vi "DC_CNTRL_select_potential.vi"(0 "Handle":u64, 1 "Ignore NACK":bool, 2 "Read Answer?":bool, 3 "Clear  RxTx Buffer?":bool, 5 "Box Number":u16(ring), 7 "Target Potential (V)":dbl, 9 "Current Potential (V)":dbl, 11 "error in (no error)":errorcluster, 12 "Max Potential (V)":dbl) -> (4 "Handle out":u64, 15 "error out":errorcluster)   [LabVIEW 2019]
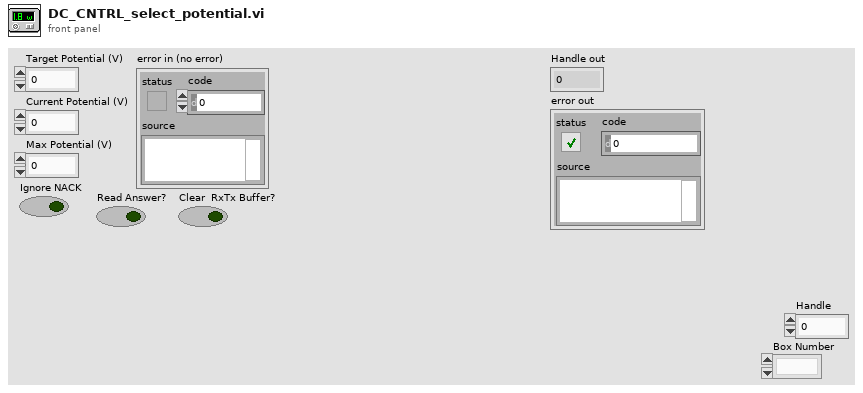
[diagram p1: front panel]
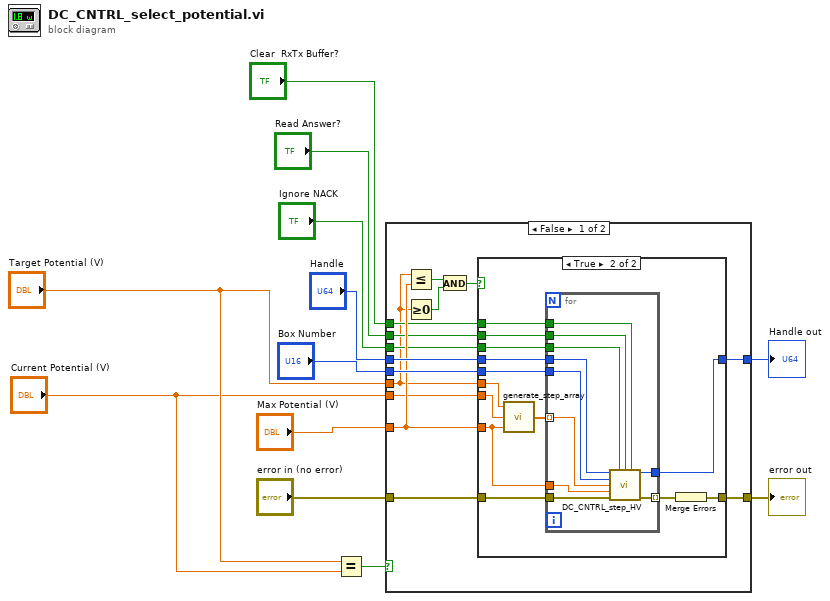
[diagram p0: block diagram]
diagram:
  n1 = Equal?(x="Target Potential (V)", y="Current Potential (V)") -> (x = y?=w12:bool)
  n2 = case shown="False" w12 {
    tunnel: "Target Potential (V)" -> [w14 _]
    tunnel: "Max Potential (V)" -> [w20 _]
    tunnel: "Handle" -> [w23 w53]
    tunnel: "Box Number" -> [w22 _]
    tunnel: "error in (no error)" -> [w21 w52]
    tunnel: "Ignore NACK" -> [w19 _]
    tunnel: "Read Answer?" -> [w18 _]
    tunnel: "Clear  RxTx Buffer?" -> [w17 _]
    tunnel: [w16 w53] -> w3
    tunnel: [w15 w52] -> w2
    tunnel: "Current Potential (V)" -> [w13 _]
    frame False {
      n3 = Less Or Equal?(x=w14, y=w20) -> (x <= y?=w25:bool)
      n4 = Greater Or Equal To 0?(x=w14) -> (x >= 0?=w24:bool)
      n5 = And(x=w25, y=w24) -> (x .and. y?=w26:bool)
      n6 = case shown="True" w26 {
        tunnel: w23 -> [w28 w41]
        tunnel: w22 -> [_ w40]
        tunnel: w21 -> [w27 w39]
        tunnel: w20 -> [_ w32]
        tunnel: w19 -> [_ w38]
        tunnel: w18 -> [_ w37]
        tunnel: w17 -> [_ w36]
        tunnel: [w28 w35] -> w16
        tunnel: [w27 w33] -> w15
        tunnel: w14 -> [_ w31]
        tunnel: w13 -> [_ w30]
        frame False {
        }
        frame True {
          n7 = call "generate_step_array.vi"("Max Potential (V)"=w32, "Current Potential (V)"=w30, "Target Potential (V)"=w31) -> ("Step Array"=w29:dbl[])
          n8 = for {
            tunnel: w41 -> [w51]
            tunnel: w40 -> [w50]
            tunnel: w39 -> [w49]
            tunnel: w32 -> [w48]
            tunnel: w38 -> [w47]
            tunnel: w37 -> [w46]
            tunnel: w36 -> [w45]
            tunnel: [w44] -> w35
            tunnel: [w43] -> w34 mode=indexing
            tunnel: w29 -> [w42] mode=indexing
            n9 = call "DC_CNTRL_step_HV.vi"("Handle"=w51, "Ignore NACK"=w47, "Read Answer?"=w46, "Clear  RxTx Buffer?"=w45, "Box Number"=w50, "Step (V)"=w42, "Max Range (V)"=w48, "error in (no error)"=w49) -> ("Handle out"=w44:u64, "error out"=w43:errorcluster)  [unwired: 6 in]
          }
          n10 = Merge Errors(w34) -> (w33:errorcluster)
        }
      }
    }
    frame True {
    }
  }
  "Handle out" <- w3
  "error out" <- w2
